vi "MeasurementServer_Event_Fire.vi"(7 "server id":i32, 8 "error in (no error)":errorcluster, 9 "status":i32, 10 "eventdata":string, 11 "gRPCid":T1) -> (0 "error out":errorcluster, 3 "gRPCid out":T1)   [LabVIEW 2019, in "labview-grpc-measurement-server.lvlib"]
uses:
  labview-grpc-measurement-server.lvlib
  MeasurementServer_gRPCid.ctl
  MeasurementServer_Event.ctl
  home/lvuser/ocv_labview_measurement_server.so
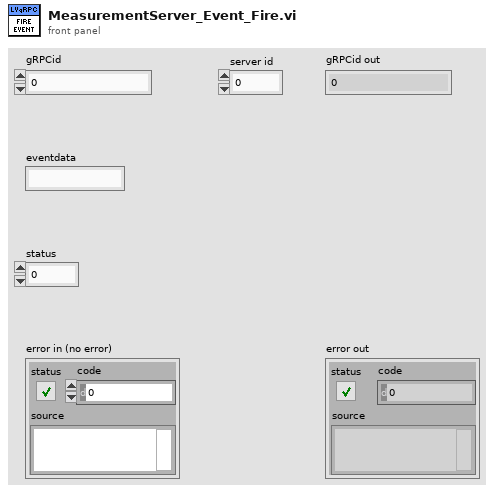
[diagram p1: front panel]
types:
  T1 = typedef "labview-grpc-measurement-server.lvlib/MeasurementServer_gRPCid.ctl" = u64
  T2 = typedef "labview-grpc-measurement-server.lvlib/MeasurementServer_Event.ctl" = cluster{"eventdata":string, "server id":i32, "status":i32}
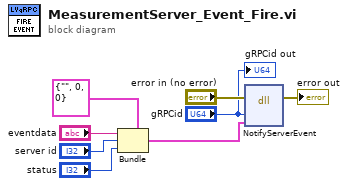
[diagram p0: block diagram]
diagram:
  n1 = Bundle(cluster=T2 {"eventdata"="", "server id"=0, "status"=0} ("ServerEvent"), "eventdata"="eventdata", "server id"="server id", "status"="status") -> (w4:T2)
  n2 = dll-call lib="home/lvuser/ocv_labview_measurement_server.so" fn="NotifyServerEvent"(error in="error in (no error)", "id"="gRPCid", "data"=w4) -> (error out=→"error out":errorcluster)  [unwired: 5 in, 1 out]
  "gRPCid out" <- "gRPCid"
